vi "mtlb simx Display Dialog.vi"(0 "clientIDandDlgTypeAndOperationMode":i32, 1 "titleColorsAndDlgColors":sgl, 5 "titleText":string, 7 "mainText":string, 9 "initialText":string, 11 "error in (no error)":errorcluster, 12 "dialogHandleAndUiHandle":i32) -> (4 "clientIDandDlgTypeAndOperationMode out":i32, 6 "function return":i32, 14 "dialogHandleAndUiHandle out":i32, 15 "error out":errorcluster)   [LabVIEW 2019, in "PXL_V-REP.lvlib"]
doc: "EXTAPI_DLLEXPORT simxInt mtlb_simxDisplayDialog(simxInt* clientIDandDlgTypeAndOperationMode,const simxChar* titleText,const simxChar* mainText,const simxChar* initialText,const simxFloat* titleColorsAndDlgColors,simxInt* dialogHandleAndUiHandle);"
uses:
  PXL_V-REP.lvlib
  <userlib>/V-REP/remoteApi.dll
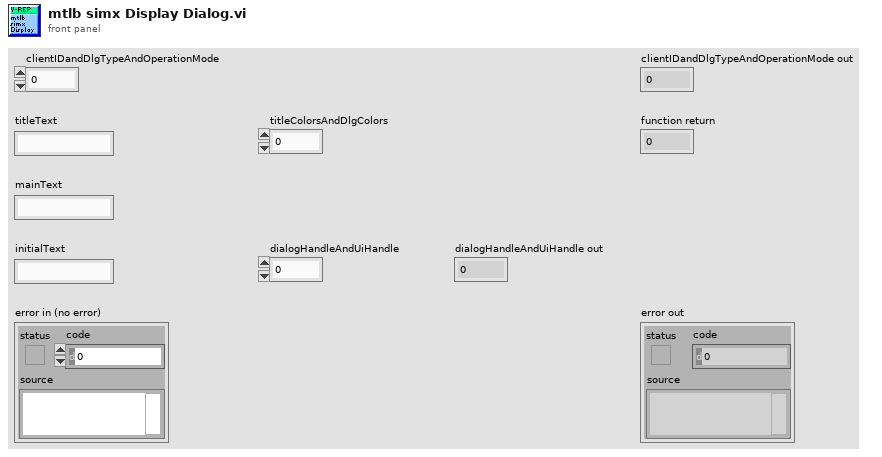
[diagram p1: front panel]
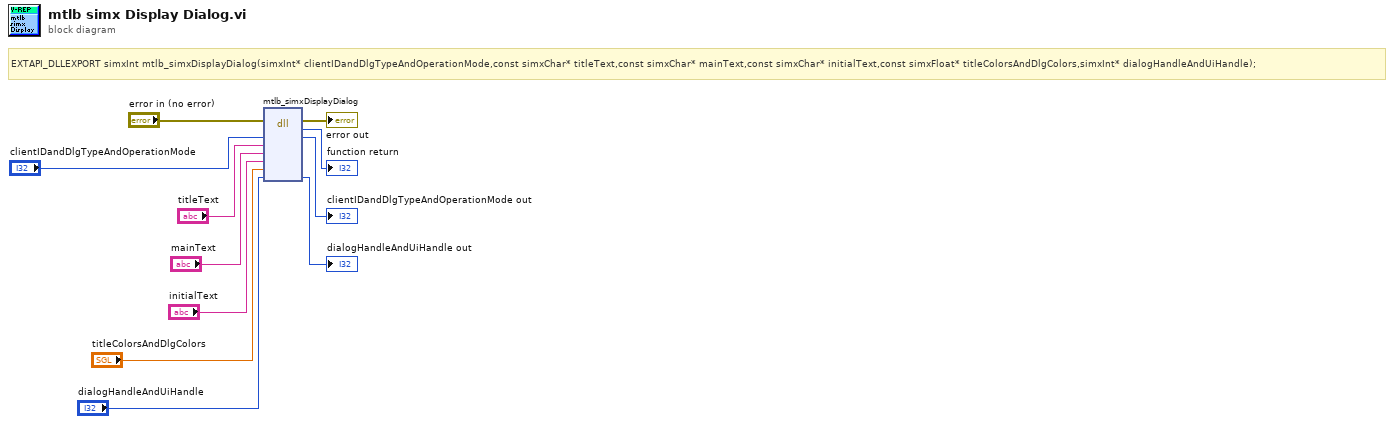
[diagram p0: block diagram]
diagram:
  # "EXTAPI_DLLEXPORT simxInt mtlb_simxDisplayDialog(simxInt* clientIDandDlgTypeAndOperationMode,const simxChar* titleText,const simxChar* mainText,const simxChar* initialText,const simxFloat* titleColorsAndDlgColors,simxInt* dialogHandleAndUiHandle);"
  n1 = dll-call lib="C:/Program Files (x86)/National Instruments/LabVIEW 2019/user.lib/V-REP/remoteApi.*" fn="mtlb_simxDisplayDialog"(error in="error in (no error)", "clientIDandDlgTypeAndOperationMode"="clientIDandDlgTypeAndOperationMode", "titleText"="titleText", "mainText"="mainText", "initialText"="initialText", "titleColorsAndDlgColors"="titleColorsAndDlgColors", "dialogHandleAndUiHandle"="dialogHandleAndUiHandle") -> (error out=→"error out":errorcluster, →"function return":i32, "clientIDandDlgTypeAndOperationMode"=→"clientIDandDlgTypeAndOperationMode out":i32, "dialogHandleAndUiHandle"=→"dialogHandleAndUiHandle out":i32)  [unwired: 6 in, 1 out]
